vi "Calc.vi"(8 "error in (no error)":errorcluster, 10 "ArrayOfWVFMs":waveform(dbl)[](array[waveform]), 11 "Max in":refnum<class "Max.lvclass">) -> (0 "error out":errorcluster, 2 "Results":string[](array[string]), 3 "Max out":refnum<class "Max.lvclass">)   [LabVIEW 2015, in "MaxLib.lvlib" / "Max.lvclass"]
uses:
  Max.lvclass
  PPL/AbstractCalcLib.lvlibp/AbstractCalc/AbstractCalc.lvclass
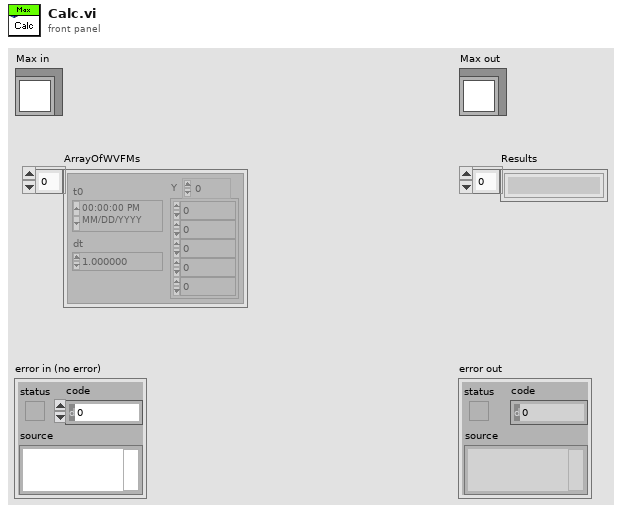
[diagram p1: front panel]
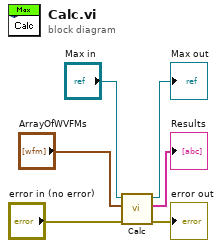
[diagram p0: block diagram]
diagram:
  n1 = call-parent "Calc.vi"("error in (no error)"="error in (no error)", "ArrayOfWVFMs"="ArrayOfWVFMs", "AbstractCalc in"="Max in") -> ("error out"=→"error out":errorcluster, "Results"=→"Results":string[], "AbstractCalc out"=→"Max out":refnum<class "Max.lvclass">)  [unwired: 6 in]
